vi "CreateCluster.vi"(8 "error in (no error)":errorcluster, 11 "DAQList in":refnum<class "DAQList.lvclass">) -> (0 "error out":errorcluster, 3 "DAQList out":refnum<class "DAQList.lvclass">)   [LabVIEW 2019, in "XCP_DaqDtoId.lvlib" / "DAQList.lvclass"]
uses:
  DAQList.lvclass
  DAQList.lvclass/DAQList.ctl
  <vilib>/ECUMC/ECUMC.llb/MC Get Prop XCP CAN IO Mode.vi
  <vilib>/ECUMC/ECUMC.llb/MC Get Prop XCP Baud Rate 64.vi
  <vilib>/ECUMC/ECUMC.llb/MC Get Prop XCP FD Baud Rate 64.vi
  <vilib>/xnet/xnet.llb/XNET Database Create (Cluster).vi
  <resource>/objmgr/xnet.rc
  <vilib>/ECUMC/ECUMC.lvlib
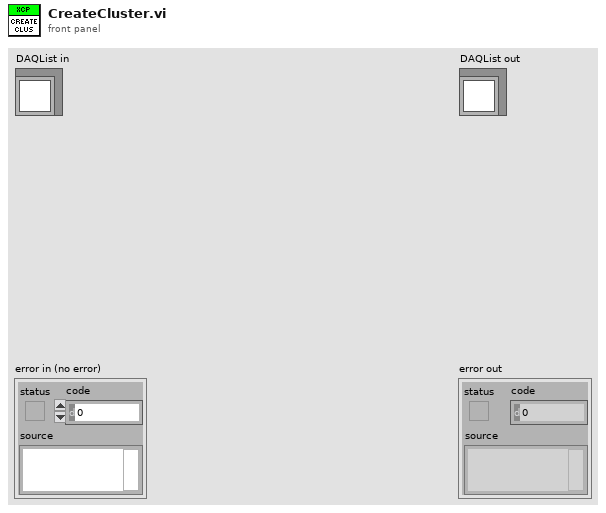
[diagram p1: front panel]
types:
  T1 = typedef "ECUMC.lvlib/MC Reference.ctt" = u32
  T2 = typedef "ECUMC.lvlib/MC CAN IO Mode.ctl" = u32
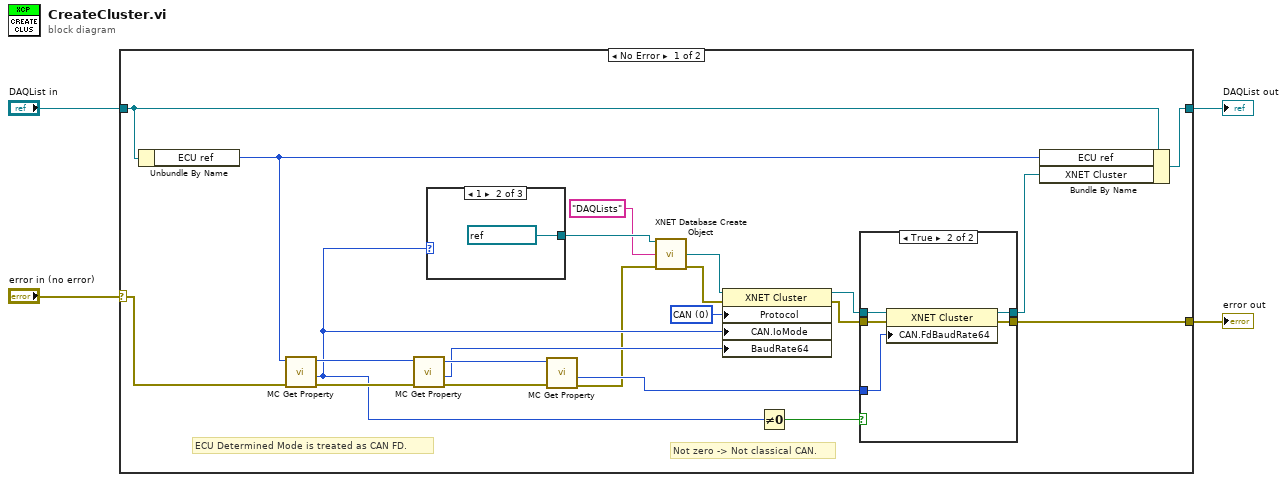
[diagram p0: block diagram]
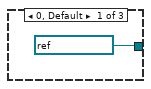
[diagram p3: hidden frame]
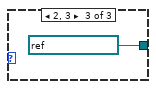
[diagram p4: hidden frame]
diagram:
  n1 = case shown="No Error" "error in (no error)" {
    selector: "error in (no error)" -> [w12 w38]
    tunnel: [w7 w38] -> w3
    tunnel: [w10 w37] -> w1
    tunnel: "DAQList in" -> [w6 w37]
    frame No Error {
      w24 = u32 0 items=["CAN", "FlexRay", "LIN"] ("Protocol")
      # "ECU Determined Mode is treated as CAN FD."
      # "Not zero -> Not classical CAN."
      n2 = Unbundle By Name(w6) -> ("ECU ref"=w8:T1)
      n3 = call-poly <vilib>:"MC Get Property.vi"("error in"=w12, "reference in"=w8) -> ("error out"=w17:errorcluster, "CAN I/O Mode"=w15:T2, "reference out"=w19:T1)  [unwired: 7 in]
      n4 = call-poly <vilib>:"MC Get Property.vi"("error in"=w17, "reference in"=w19) -> ("error out"=w16:errorcluster, "XCP Baud Rate 64"=w14:u64, "reference out"=w18:T1)  [unwired: 7 in]
      n5 = case shown="1" w15 {
        tunnel: [refnum<k21> ":memory:" ("database in (:memory:)") refnum<k21> ":can_fd:" ("database in (:memory:)") refnum<k21> ":can_fd_brs:" ("database in (:memory:)")] -> w23
        frame 0, Default {
        }
        frame 1 {
        }
        frame 2, 3 {
        }
      }
      n6 = call-poly <vilib>:"MC Get Property.vi"("error in"=w16, "reference in"=w18) -> ("error out"=w11:errorcluster, "XCP FD Baud Rate 64"=w13:u64)  [unwired: 7 in, 1 out]
      n7 = call-poly <vilib>:"XNET Database Create Object.vi"("database in"=w23, "cluster name"="DAQLists" ("Cluster Name"), "error in (no error)"=w11) -> ("cluster out"=w25:refnum<k21>, "error out"=w26:errorcluster)  [unwired: 10 in, 1 out]
      n8 = property class="XNET Cluster"(reference=w25, error in=w26, "Protocol"=w24, "CAN.IoMode"=w15, "BaudRate64"=w14) -> (reference out=w22:refnum<k21>, error out=w21:errorcluster)
      n9 = Not Equal To 0?(x=w15) -> (x != 0?=w20:bool)
      n10 = case shown="True" w20 {
        tunnel: w22 -> [w28 w33]
        tunnel: w21 -> [w27 w32]
        tunnel: [w27 w31] -> w7
        tunnel: [w28 w30] -> w9
        tunnel: w13 -> [_ w29]
        frame False {
        }
        frame True {
          n11 = property class="XNET Cluster"(reference=w33, error in=w32, "CAN.FdBaudRate64"=w29) -> (reference out=w30:refnum<k21>, error out=w31:errorcluster)
        }
      }
      n12 = Bundle By Name(cluster=w6, "ECU ref"=w8, "XNET Cluster"=w9) -> (w10:refnum<class "DAQList.lvclass">)
    }
    frame Error {
    }
  }
  "error out" <- w3
  "DAQList out" <- w1
